vi "Check for Included Angle (array).vi"(6 "coerce angle":bool, 7 "angle units":T2 items=["radian in, radian out", "radian in, degree out", "degree in, degree out", "degree in, radian out"], 8 "output angle range":T1=1 items=["none", "-180 to 180 (-pi to pi)", "0 to 360 (0 to 2pi)"], 9 "End Angle":dbl[](array[numeric]), 10 "Start Angle":dbl[](array[numeric]), 11 "Angle In":dbl[](array[numeric])) -> (0 "error":i32, 2 "In Range?":bool[](array[boolean]), 3 "Angle Out":dbl[](array[numeric]))   [LabVIEW 2017, in "NI_AAL_Angle.lvlib"]
doc: "Checks whether one or multiple input angles are within the counterclockwise range.\n\nWire data to any of the angle inputs to determine the polymorphic instance to use or manually select the instance."
uses:
  <vilib>/Analysis/NI_AAL_Angle.lvlib
  <vilib>/Analysis/coordinate.llb/Angle Units.ctl
  <vilib>/Analysis/coordinate.llb/Angle Range (Degree).ctl
  <vilib>/Analysis/coordinate.llb/Wrap Angle (scalar).vi
  <vilib>/Analysis/coordinate.llb/Absolute Angle Difference (scalar).vi
  <vilib>/Analysis/coordinate.llb/Set Angle Unit.vi
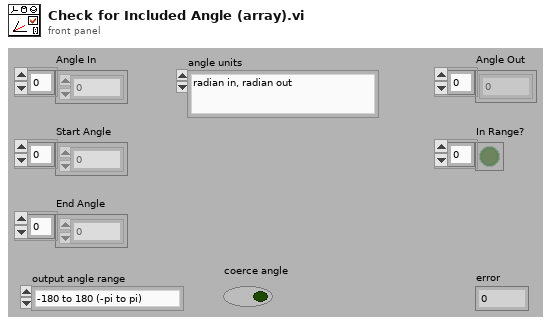
[diagram p1: front panel]
types:
  T1 = typedef "NI_AAL_Angle.lvlib/Angle Range (Degree).ctl" = u16
  T2 = typedef "NI_AAL_Angle.lvlib/Angle Units.ctl" = i32
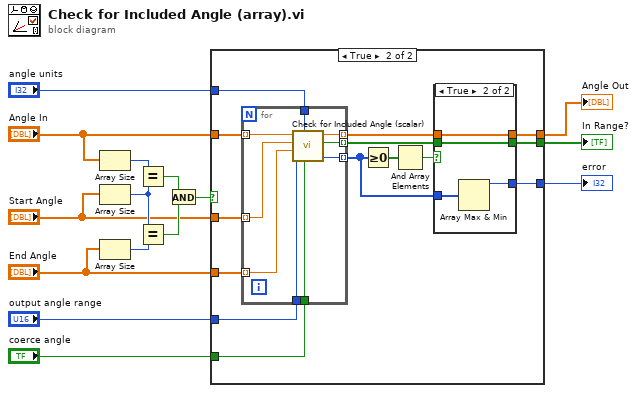
[diagram p0: block diagram]
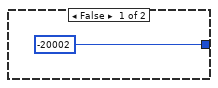
[diagram p2: hidden frame]
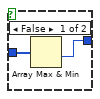
[diagram p3: hidden frame]
diagram:
  n1 = Array Size(array="Angle In") -> (size(s)=w15:i32)
  n2 = Array Size(array="Start Angle") -> (size(s)=w14:i32)
  n3 = Array Size(array="End Angle") -> (size(s)=w13:i32)
  n4 = Equal?(x=w15, y=w14) -> (x = y?=w12:bool)
  n5 = Equal?(x=w14, y=w13) -> (x = y?=w11:bool)
  n6 = And(x=w12, y=w11) -> (x .and. y?=w10:bool)
  n7 = case shown="True" w10 {
    tunnel: "Angle In" -> [_ w30]
    tunnel: "Start Angle" -> [_ w29]
    tunnel: "angle units" -> [_ w28]
    tunnel: "End Angle" -> [_ w27]
    tunnel: [_ w23] -> w3
    tunnel: [-20002 w21] -> w1
    tunnel: "output angle range" -> [_ w20]
    tunnel: "coerce angle" -> [_ w19]
    tunnel: [_ w17] -> w2
    frame False {
    }
    frame True {
      n8 = for {
        tunnel: w30 -> [w44] mode=indexing
        tunnel: w29 -> [w43] mode=indexing
        tunnel: w28 -> [w45]
        tunnel: w27 -> [w42] mode=indexing
        tunnel: [w39] -> w24 mode=indexing
        tunnel: [w37] -> w22 mode=indexing
        tunnel: w20 -> [w41]
        tunnel: w19 -> [w40]
        tunnel: [w38] -> w18 mode=indexing
        n9 = call <vilib>:"Check for Included Angle (scalar).vi"("coerce angle"=w40, "angle units"=w45, "output angle range"=w41, "end angle"=w42, "start angle"=w43, "angle in"=w44) -> ("error"=w37:i32, "in range?"=w38:bool, "angle out"=w39:dbl)  [unwired: 3 in]
      }
      n10 = Greater Or Equal To 0?(x=w22) -> (x >= 0?=w26:bool[])
      n11 = And Array Elements(Boolean array=w26) -> (logical AND=w25:bool)
      n12 = case shown="True" w25 {
        tunnel: w24 -> [_ w36]
        tunnel: [_ w36] -> w23
        tunnel: w22 -> [w32 w35]
        tunnel: [w31 w34] -> w21
        tunnel: w18 -> [_ w33]
        tunnel: [_ w33] -> w17
        frame False {
          n13 = Array Max & Min(array=w32) -> (min value=w31:i32)  [unwired: 3 out]
        }
        frame True {
          n14 = Array Max & Min(array=w35) -> (max value=w34:i32)  [unwired: 3 out]
        }
      }
    }
  }
  "error" <- w1
  "Angle Out" <- w3
  "In Range?" <- w2
